vi "Sample Code.vi"() -> ()   [LabVIEW 2025]
uses:
  Tdef/Product enum.ctl
  Abstract License/Software License Manager.lvclass
  SW License Manager.lvlib
panel:
  in  "Product":T1
  out "ok?":bool
  out "Body":string
  in  "Company_Info":T2
  out "Check ok?":bool
  in  "Proccess":T3(ring)=enum."Check"
  # "1. Select Proccess\n2. Modified Product Reference enum\n3. Add Company_Info to create a new license"
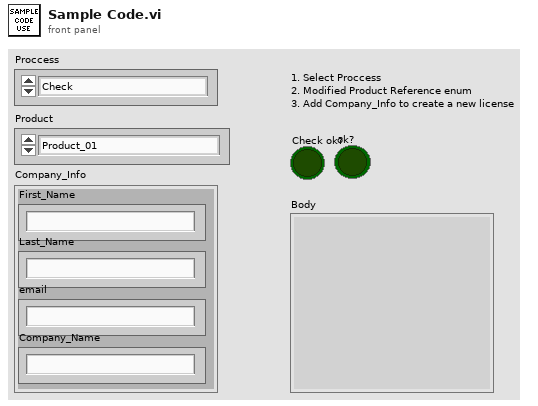
[diagram p1: front panel]
types:
  T1 = typedef "SW License Manager.lvlib/Product enum.ctl" = enum16{"Product_01", "Product_02", "Product_03"}
  T2 = cluster{"First_Name":string, "Last_Name":string, "email":string, "Company_Name":string}
  T3 = enum16{"Create", "Activate", "Deactivate", "Check"}
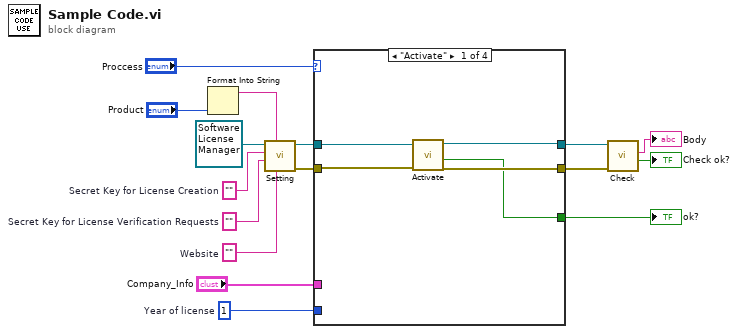
[diagram p0: block diagram]
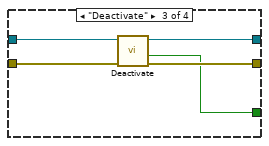
[diagram p3: hidden frame]
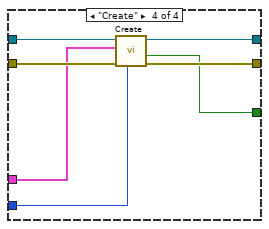
[diagram p4: hidden frame]
diagram:
  w2 = 1  # Year of license
  w7 = ""  # Secret Key for License Creation
  w8 = ""  # Secret Key for License Verification Requests
  w9 = ""  # Website
  n1 = Format Into String("Product") -> (resulting string=w5:string)  [unwired: 3 in, 1 out]
  n2 = call-dynamic "Setting.vi"("Website"=w9, "Product_Ref"=w5, "Secret Key for License Verification Requests"=w8, "Secret Key for License Creation"=w7, "object License in"=refnum<class "Software License Manager.lvclass"> refnum ("Abstract License.lvclass")) -> ("error out"=w13:errorcluster, "Object License out"=w14:refnum<class "Software License Manager.lvclass">)  [unwired: 5 in]
  n3 = case shown="\"Activate\"" "Proccess" {
    tunnel: w14 -> [w21 w23 w28 w29]
    tunnel: w13 -> [w18 w22 w27 w33]
    tunnel: [w20 w23 w26 w34] -> w12
    tunnel: [w19 w22 w25 w35] -> w11
    tunnel: [w17 _ w24 w32] -> w4
    tunnel: w2 -> [_ _ _ w31]
    tunnel: "Company_Info" -> [_ _ _ w30]
    frame "Activate" {
      n4 = call-dynamic "Activate.vi"("error in (no error)"=w18, "Object License in"=w21) -> ("error out"=w19:errorcluster, "ok?"=w17:bool, "Object License out"=w20:refnum<class "Software License Manager.lvclass">)  [unwired: 7 in]
    }
    frame "Check", Default {
    }
    frame "Deactivate" {
      n5 = call-dynamic "Deactivate.vi"("error in (no error)"=w27, "Object License in"=w28) -> ("error out"=w25:errorcluster, "ok?"=w24:bool, "Object License out"=w26:refnum<class "Software License Manager.lvclass">)  [unwired: 7 in]
    }
    frame "Create" {
      n6 = call-dynamic "Create.vi"("Year of license"=w31, "error in (no error)"=w33, "Company_Info"=w30, "Object License Manager in"=w29) -> ("error out"=w35:errorcluster, "ok?"=w32:bool, "Object License Manager out"=w34:refnum<class "Software License Manager.lvclass">)  [unwired: 5 in]
    }
  }
  "ok?" <- w4
  n7 = call-dynamic "Check.vi"("error in (no error)"=w11, "Object License Manager in"=w12) -> ("ok?"=→"Check ok?":bool, "Body"=→"Body":string)  [unwired: 6 in, 2 out]
